vi "Ejercicio_08_strings.vi"() -> ()   [LabVIEW 2020]
panel:
  out "output 1":dbl
  out "after substring":string
  out "match substring":string
  out "before substring":string
  out "offset past match":i32
  in  "input 1":dbl
  in  "Unidades":string="Volts"
  out "Longitud":i32
  in  "Encabezado":string="El valor de voltaje es "
  out "concatenated string":string
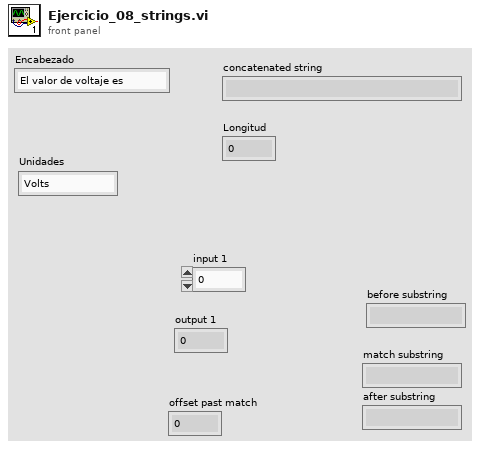
[diagram p1: front panel]
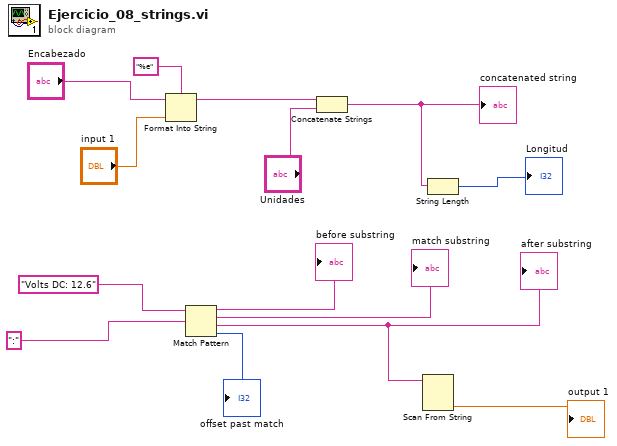
[diagram p0: block diagram]
diagram:
  n1 = Format Into String "Format Into String"(format string="%e", initial string="Encabezado", "input 1") -> (resulting string=w12:string)  [unwired: 1 in, 1 out]
  n2 = Match Pattern(string="Volts DC: 12.6", regular expression=":") -> (before substring=→"before substring":string, match substring=→"match substring":string, after substring=w2:string, offset past match=→"offset past match":i32)  [unwired: 1 in]
  "after substring" <- w2
  n3 = Concatenate Strings "Concatenate Strings"(w12, "Unidades") -> (w11:string)
  "concatenated string" <- w11
  n4 = Scan From String "Scan From String"(input string=w2) -> (output 1=→"output 1":dbl)  [unwired: 4 in, 3 out]
  n5 = String Length(string=w11) -> (length=→"Longitud":i32)
